vi "niScope EX Getting Started.vi"(0 "Channel(s)":string="0", 1 "resource name":refnum<k15>="Dev1" caption="Resource Name(s)", 2 "Simulate?":bool) -> (27 "Waveform Graph":T1(graph))   [LabVIEW 2021, in "niScope EX Getting Started dependencies.lvlib"]
doc: "Example: Getting Started\n\nRecommended Input Signal: 100 kHz, 1.8 Vpp, sine wave\n\nDevices Supported: Refer to NI Example Finder\n\nLabVIEW Description:\n\nThis example opens a session to the NI-SCOPE driver by passing in the device's resource name to the Initialize VI. The resource name is a unique identifier for your National Instruments' hardware product. It can be found (and changed) by running Measurement & Automation Explorer (MAX). A shortcut to MAX is placed on your desktop when NI-SCOPE or NI-DAQ is installed.\n\nThe session handle returned from the Initialize VI is a parameter to all VIs in the NI-SCOPE driver. Only one session may be opened at a time for your oscilloscope, and every session should be closed by calling the Close vi. The session should be closed even when an error occurs.\n\nThe Auto Setup VI takes several acquisitions to measure the amplitude and frequency of the input signal. This allows it to optimally set properties such as the sample rate, vertical range, and minimum record length. The Read VI, initiates an acquisition, waits for it to finish, and fetches the data from the oscilloscope. The data is returned as a bundle of the initial x, x increment, and waveform. Initial x is the time of the first point in the waveform relative to the trigger, while the x increment is the time between two points in the waveform. This bundle may be directly wired to a waveform graph, to display the waveform with timing information. \n\nThe Error Handler VI translates any error messages into text messages."
uses:
  niScope EX Getting Started dependencies.lvlib
  <instrlib>/niScope/Acquire/niScope Multi Read Cluster.vi
panel:
  # "Overview: Demonstrates the minimal code needed to use NI-SCOPE.\nRequirements: NI-SCOPE\nInstructions: \n1.  Select the appropriate device in the Resource Name control.\n2.  Enter the channels you would like to acquire from in the Channel(s) control.\n3.  Run the VI."
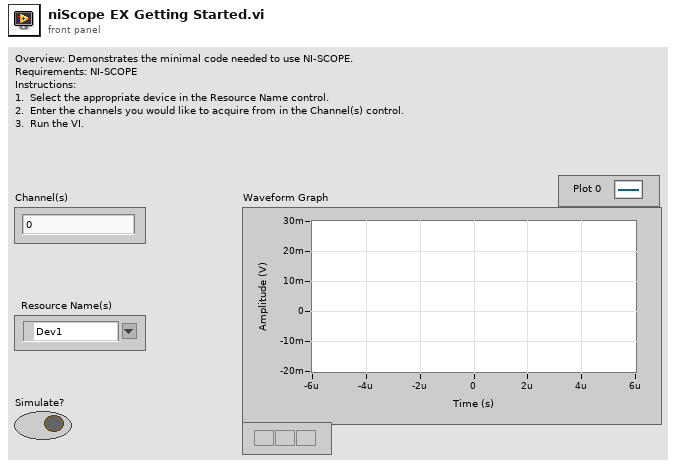
[diagram p1: front panel]
types:
  T1 = cluster{"relativeInitialX":dbl, "xIncrement":dbl, "wfm":dbl[]}[]
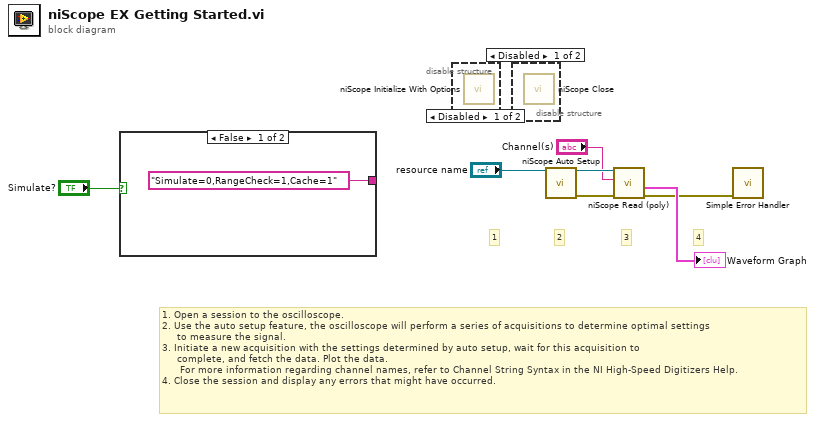
[diagram p0: block diagram]
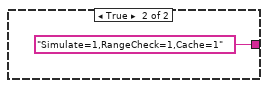
[diagram p4: hidden frame]
diagram:
  # "1. Open a session to the oscilloscope.\n2. Use the auto setup feature, the oscilloscope will perform a series of acquisitions to determine optimal settings\n     to measure the signal.\n3. Initiate a new acquisition with the settings determined by auto setup, wait for this acquisition to\n     complete, and fetch the data. Plot the data.\n      For more information regarding channel names, refer to Channel String Syntax in the NI High-Speed Digitizers Help.\n4. Close the session and display any errors that might have occurred."
  # "4"
  # "3"
  # "2"
  # "1"
  n1 = case shown="False" "Simulate?" {
    tunnel: ["Simulate=0,RangeCheck=1,Cache=1" ("option string") "Simulate=1,RangeCheck=1,Cache=1" ("option string")] -> _
    frame False {
    }
    frame True {
    }
  }
  n2 = disable-structure shown="Disabled" {
    frame Disabled {
      n3 = call <instrlib>:"niScope Initialize With Options.vi"() -> ()  [unwired: 14 in, 2 out]
    }
    frame Enabled {
    }
  }
  n4 = disable-structure shown="Disabled" {
    frame Disabled {
      n5 = call <instrlib>:"niScope Close.vi"() -> ()  [unwired: 15 in, 1 out]
    }
    frame Enabled {
    }
  }
  n6 = call <instrlib>:"niScope Auto Setup.vi"("instrument handle"="resource name") -> ("instrument handle out"=w7:refnum<k15>, "error out"=w6:errorcluster)  [unwired: 13 in]
  n7 = call-poly <instrlib>:"niScope Read (poly).vi"("error in"=w6, "channels"="Channel(s)", "instrument handle"=w7) -> ("error out"=w3:errorcluster, "waveform"=→"Waveform Graph":T1)  [unwired: 5 in, 2 out]
  n8 = call <vilib>:"Simple Error Handler.vi"("error in (no error)"=w3) -> ()  [unwired: 4 in, 5 out]
